vi "Read Version.vi"(8 "error in (no error)":errorcluster, 11 "csv-formatter Config in":refnum<class "csv-formatter Config.lvclass">) -> (0 "error out":errorcluster, 2 "Version":string, 3 "csv-formatter Config out":refnum<class "csv-formatter Config.lvclass">)   [LabVIEW 2015, in "csv-formatter Config.lvclass"]
uses:
  csv-formatter Config.lvclass
  csv-formatter Config.lvclass/csv-formatter Config.ctl
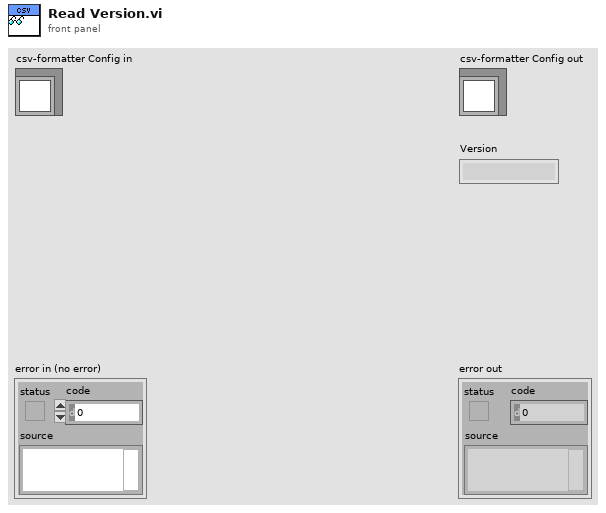
[diagram p1: front panel]
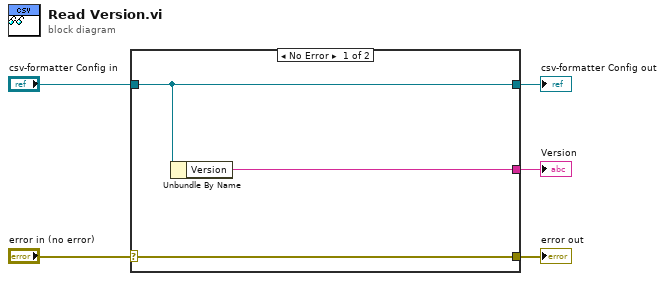
[diagram p0: block diagram]
diagram:
  n1 = case shown="No Error" "error in (no error)" {
    selector: "error in (no error)" -> [w8 w9]
    tunnel: [w8 w9] -> w4
    tunnel: [w7 w10] -> w2
    tunnel: "csv-formatter Config in" -> [w7 w10]
    tunnel: [w6 _] -> w1
    frame No Error {
      n2 = Unbundle By Name(w7) -> ("Version"=w6:string)
    }
    frame Error {
    }
  }
  "error out" <- w4
  "csv-formatter Config out" <- w2
  "Version" <- w1
